vi "Add Routine.vi"(8 "error in (no error)":errorcluster, 11 "Node Ptr":u64 format="%.0x") -> (0 "error out":errorcluster)   [LabVIEW 2015, in "Diagnostics Addon System Explorer.lvlib"]
uses:
  Diagnostics Addon System Explorer.lvlib
  Shared/Types/Routine Paramaters.ctl
  Shared/Types/Input and Output Signal Parameters.ctl
  Shared/Types/Signal Parameters.ctl
  <vilib>/NI Veristand/Custom Device API/Custom Device API.lvlib
  <vilib>/NI Veristand/Custom Device Tools/Custom Device Utility Library/Custom Device Utility Library.lvlib
  Shared/Diagnostics Addon Shared.lvlib
panel:
  in  "Tag":string
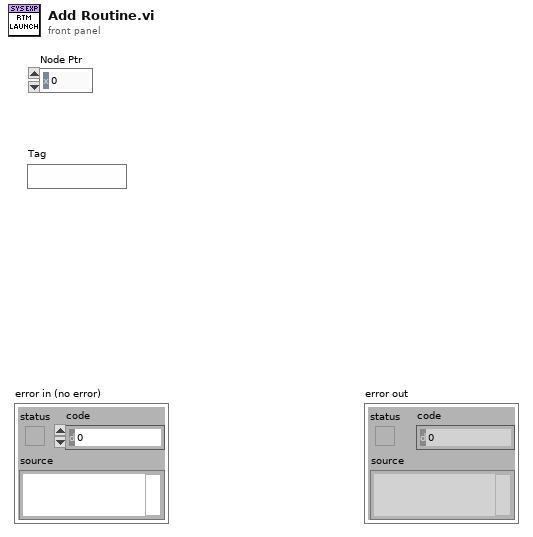
[diagram p1: front panel]
types:
  T1 = typedef "Custom Device API.lvlib/Custom Device Item Ref.ctl" = u64
  T2 = typedef "Custom Device API.lvlib/Custom Device Item Info.ctl" = cluster{"Name":string, "Is Channel":bool, "GUID":string, "Is Waveform":bool}
  T3 = typedef "Diagnostics Addon Shared.lvlib/Routine Paramaters.ctl" = cluster{"Name":string, "Description":string, "ID":u16, "Start Parameters":T4, "Request Parameters":T4, "Stop Parameters":T4}
  T4 = typedef "Diagnostics Addon Shared.lvlib/Input and Output Signal Parameters.ctl" = cluster{"Cmd":T5[], "Response":T5[]}
  T5 = typedef "Diagnostics Addon Shared.lvlib/Signal Parameters.ctl" = cluster{"Start Bit":u8, "Length":u8, "Scaling Factor":dbl, "Scaling Offset":dbl, "Minimum":dbl, "Maximum":dbl, "Data Type":u32, "Byte Order":u32, "Default Value":dbl, "Name":string, "Units":string, "Description":string}
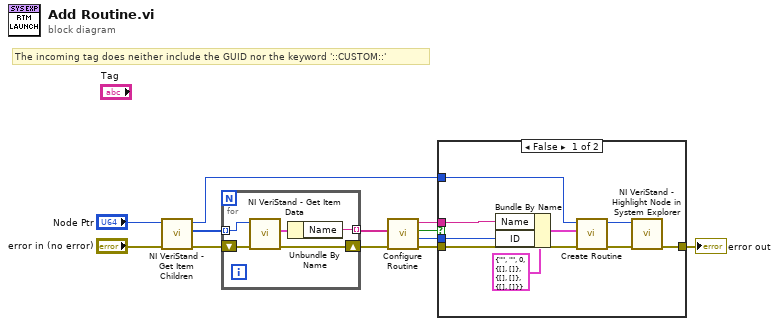
[diagram p0: block diagram]
diagram:
  # "The incoming tag does neither include the GUID nor the keyword '::CUSTOM::'"
  n1 = call <vilib>:"NI VeriStand - Get Item Children.vi"("error in (no error)"="error in (no error)", "Item Ref in"="Node Ptr") -> ("error out"=w10:errorcluster, "Child Refs"=w8:T1[], "Item Ref out"=w7:T1)  [unwired: 6 in, 1 out]
  n2 = for {
    tunnel: [w15] -> w6 mode=indexing
    shift-right: [w14] -> w5
    shift-left: w10 -> [w16]
    tunnel: w8 -> [w13] mode=indexing
    n3 = call <vilib>:"NI VeriStand - Get Item Data.vi"("error in (no error)"=w16, "Item Ref in"=w13) -> ("error out"=w14:errorcluster, "Item Info"=w17:T2)  [unwired: 8 out]
    n4 = Unbundle By Name(w17) -> ("Name"=w15:string)
  }
  n5 = call "Configure Routine.vi"("error in (no error)"=w5, "Existing PIDs"=w6) -> ("error out"=w4:errorcluster, "ID out"=w3:u16, "Cancel PID?"=w2:bool, "Name out"=w1:string)  [unwired: 6 in]
  n6 = case shown="False" w2 {
    tunnel: w4 -> [w25 w27]
    tunnel: w7 -> [w22 _]
    tunnel: w1 -> [w19 _]
    tunnel: [w26 w27] -> w9
    tunnel: w3 -> [w18 _]
    frame False {
      n7 = Bundle By Name(cluster=T3 {"Name"="", "Description"="", "ID"=0, "Start Parameters"={"Cmd"=[], "Response"=[]}, "Request Parameters"={"Cmd"=[], "Response"=[]}, "Stop Parameters"={"Cmd"=[], "Response"=[]}} ("Routine"), "Name"=w19, "ID"=w18) -> (w20:T3)
      n8 = call "Create Routine.vi"("error in (no error)"=w25, "Routine"=w20, "Section Ptr"=w22) -> ("error out"=w24:errorcluster, "Parent Ref out"=w23:T1)  [unwired: 7 in]
      n9 = call <vilib>:"NI VeriStand - Highlight Node in System Explorer.vi"("error in (no error)"=w24, "Item Ref in"=w23) -> ("error out"=w26:errorcluster)  [unwired: 8 in, 1 out]
    }
    frame True {
    }
  }
  "error out" <- w9
